vi "FOR LOOP  USING ARRAYS.vi"() -> ()   [LabVIEW 2018]
panel:
  out "Array 3":i32[](array[numeric])
  out "INDEXING WITH CONDITION":dbl[](array[numeric])
  out "number: 0 to 1":dbl
  out "Array 4":dbl[](array[numeric])
  in  "Array 2":i32[](array[numeric])
  out "Numeric 2":i32
  out "Numeric":i32
  in  "Array":i32[](array[numeric])
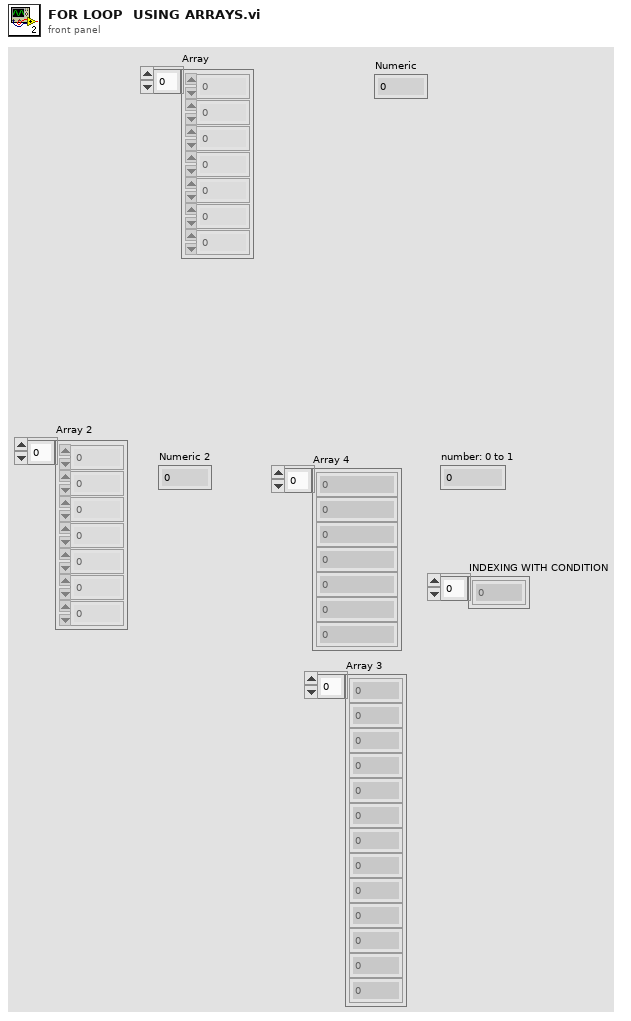
[diagram p1: front panel]
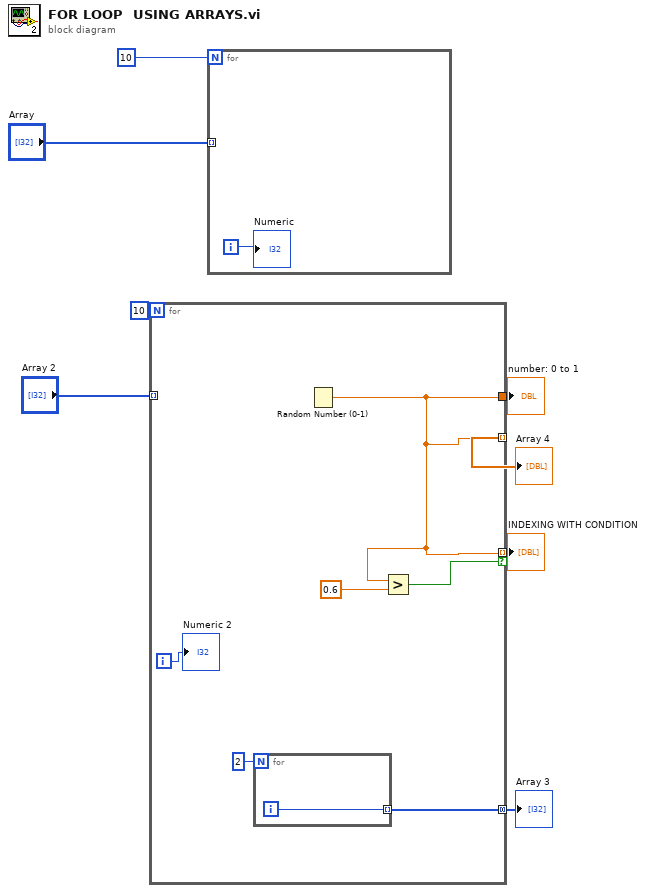
[diagram p0: block diagram]
diagram:
  n1 = for {
    N: 10 -> [_]
    tunnel: "Array 2" -> [_] mode=indexing
    tunnel: [w12] -> w4 mode=indexing
    tunnel: [w12] -> w3
    tunnel: [w12] -> w2 mode=indexing if=w13
    tunnel: [w9] -> w1 mode=concatenating
    i -> [w14]
    n2 = for {
      N: 2 -> [_]
      tunnel: [w15] -> w9 mode=indexing
      i -> [w15]
    }
    n3 = Random Number (0-1)() -> (number: 0 to 1=w12:dbl)
    n4 = Greater?(x=w12, y=0.6) -> (0:w13:bool)
    "Numeric 2" <- w14
  }
  "Array 4" <- w4
  "number: 0 to 1" <- w3
  "INDEXING WITH CONDITION" <- w2
  "Array 3" <- w1
  n5 = for {
    N: 10 -> [_]
    tunnel: "Array" -> [_] mode=indexing
    i -> [w16]
    "Numeric" <- w16
  }
